vi "FL Create Membership Function (Gaussian).vi"(0 "left base":dbl, 1 "name":string, 5 "left top":dbl, 7 "right top":dbl, 9 "right base":dbl, 11 "error in (no error)":errorcluster, 12 "color":u32(colorbox)) -> (4 "membership function":T1 {"shape" items=["Triangle", "Trapezoid", "Singleton", "Sigmoid", "Gaussian", "User-Defined"]}, 15 "error out":errorcluster)   [LabVIEW 2020, in "NI_Fuzzy_Logic_API.lvlib"]
doc: "Creates a membership function for a linguistic variable. You also can use the Define Variable dialog box to create membership functions interactively."
uses:
  <vilib>/addons/Fuzzy Logic/NI_Fuzzy_Logic_API.lvlib
  <vilib>/addons/Fuzzy Logic/TypeDefs/FL Membership Function.ctl
  <vilib>/addons/Fuzzy Logic/TypeDefs/FL Membership Function Shape.ctl
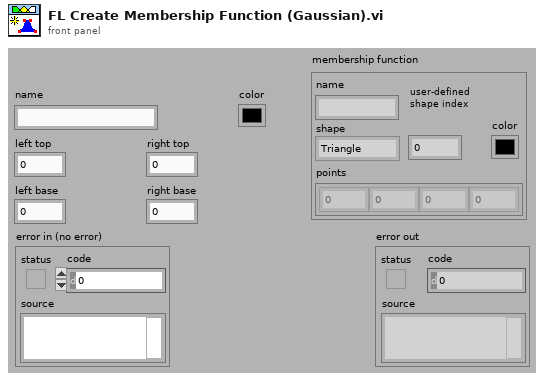
[diagram p1: front panel]
types:
  T1 = typedef "NI_Fuzzy_Logic_API.lvlib/FL Membership Function.ctl" = cluster{"name":string, "shape":T2, "points":dbl[], "color":u32, "user-defined shape index":i32}
  T2 = typedef "NI_Fuzzy_Logic_API.lvlib/FL Membership Function Shape.ctl" = u16
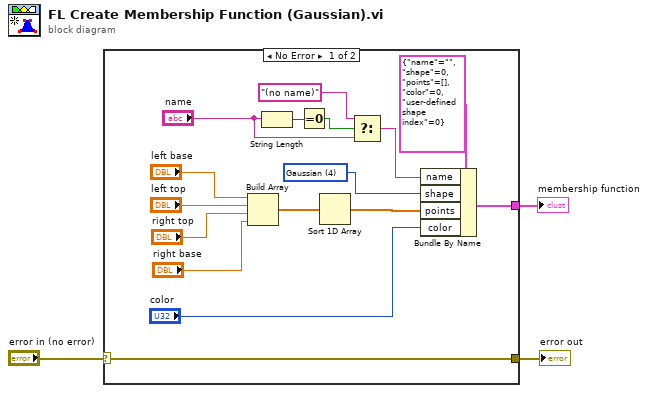
[diagram p0: block diagram]
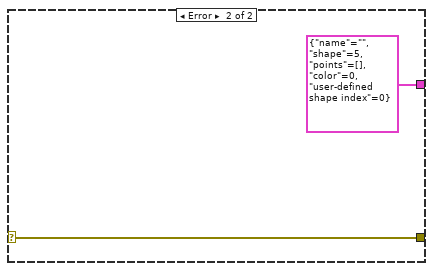
[diagram p2: hidden frame]
diagram:
  n1 = case shown="No Error" "error in (no error)" {
    selector: "error in (no error)" -> [w11 w21]
    tunnel: [w19 T1 {"name"="", "shape"=5, "points"=[], "color"=0, "user-defined shape index"=0} ("Membership Function")] -> w1
    tunnel: [w11 w21] -> w2
    frame No Error {
      w4 = T2 4 items=["Triangle", "Trapezoid", "Singleton", "Sigmoid", "Gaussian", "User-Defined"] ("shape")
      n2 = Build Array("left base", "left top", "right top", "right base") -> (w12:dbl[])
      n3 = String Length(string="name") -> (length=w18:i32)
      n4 = Equal To 0?(x=w18) -> (x = 0?=w17:bool)
      n5 = Sort 1D Array(array=w12) -> (sorted array=w8:dbl[])
      n6 = Select(t="(no name)", s=w17, f="name") -> (s? t:f=w7:string)
      n7 = Bundle By Name(cluster=T1 {"name"="", "shape"=0, "points"=[], "color"=0, "user-defined shape index"=0} ("Membership Function"), "name"=w7, "shape"=w4, "points"=w8, "color"="color") -> (w19:T1)
    }
    frame Error {
    }
  }
  "membership function" <- w1
  "error out" <- w2
